vi "BoardClassType.vi"(8 "error in (no error)":errorcluster, 11 "Software License Manager in":refnum<class "Software License Manager.lvclass">) -> (0 "error out":errorcluster, 2 "Board":refnum<class "Board.lvclass">, 3 "Software License Manager out":refnum<class "Software License Manager.lvclass">)   [LabVIEW 2025, in "SW License Manager.lvlib" / "Software License Manager.lvclass"]
doc: "Plugin board class Overide as needed"
uses:
  Software License Manager.lvclass
  Board/Board.lvclass
  Board_classes/Motherboard/Motherboard.lvclass
  C:/Users/Avern/Documents/Software/Software-License-Manager/Code/Board/Board.lvclass
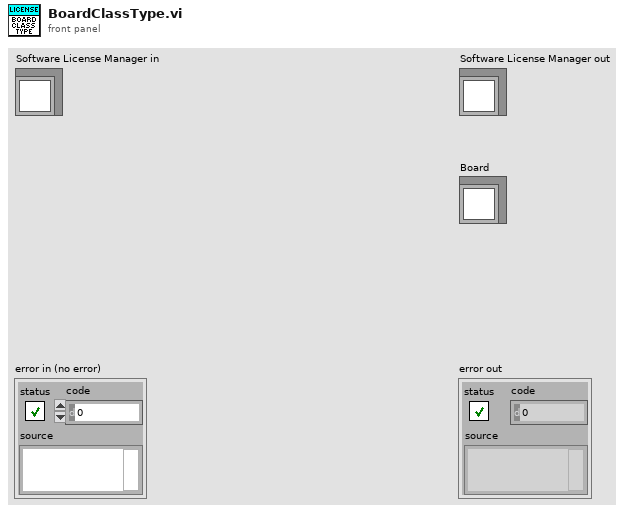
[diagram p1: front panel]
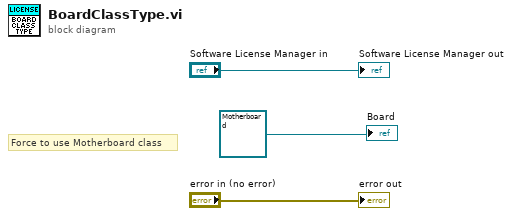
[diagram p0: block diagram]
diagram:
  # "Force to use Motherboard class"
  "error out" <- "error in (no error)"
  "Software License Manager out" <- "Software License Manager in"
  "Board" <- refnum<class "Motherboard.lvclass"> refnum ("License Manager Wordpress.lvlib:Motherboard.lvclass")
